vi "RSMA Receiver - 1 Channel 16QAM.vi"() -> ()   [LabVIEW 2022 SP3]
panel:
  out "Decoded message 2":string
  out "Acc. BER 2":dbl format="%#_4g"
  out "No. Bits 2":dbl format="%#_6f"
  out "Inst. BER 2":dbl format="%#_4g"
  out "Acum. Err 2":dbl
  in  "Expected message 2":string="rmod tempor invidunt ut labore et dolore magna aliquyam erat, sed diam volu"
  out "Number of bits":dbl[](array[numeric])
  out "Accuracy error":dbl[](array[numeric])
  out "Accumulated error":dbl[](array[numeric])
  out "Iterations":dbl format="%#_4g"
  out "Decoded message":string
  out "Constellation Map":cdb[](graph)
  in  "Decode M2?":bool
  in  "Tab Control":enum32{"USRP Parameters", "Rx Info", "BER"}(tab)
  in  "USRP ControledParameters":T1={"Active Antenna"="RX2", "Gain (dB)"=0.0, "Carrier Frequency"=2400000000.0, "IQ Rate"=2000000.0, "Active channels"="0"} {"IQ Rate" format="%#_6p"; "Carrier Frequency" format="%#_6p"; "Gain (dB)" format="%#_6f"}
  in  "Device selection":refnum<k15>="RIO0"
  in  "Trigger level":dbl=0.01 format="%f"
  out "?":T2
  out "SIG valid?":bool
  out "Frequency offset":dbl
  out "Coerced Parameters":T3={"IQ Rate"=100000.0, "Carrier  Freq."=100000.0, "Gain"=0.0} {"Gain" format="%#_6f"; "Carrier  Freq." format="%#_6p"; "IQ Rate" format="%#_6p"}
  out "Error out":errorcluster
  in  "Expected message":string="Lorem ipsum dolor sit amet, consetetur sadipscing elitr, sed diam nonumy eirmod tempor invidunt ut labore et dolore magna aliquyam erat, sed diam volu"
  in  "Record BER":bool
  in  "Refresh Button":bool
  out "Inst. BER":dbl format="%#_4g"
  out "No. Bits":dbl format="%#_6f"
  out "Acum. Err":dbl
  out "Acc. BER":dbl format="%#_4g"
  in  "error in (no error)":errorcluster
  # "RSMA Reciever"
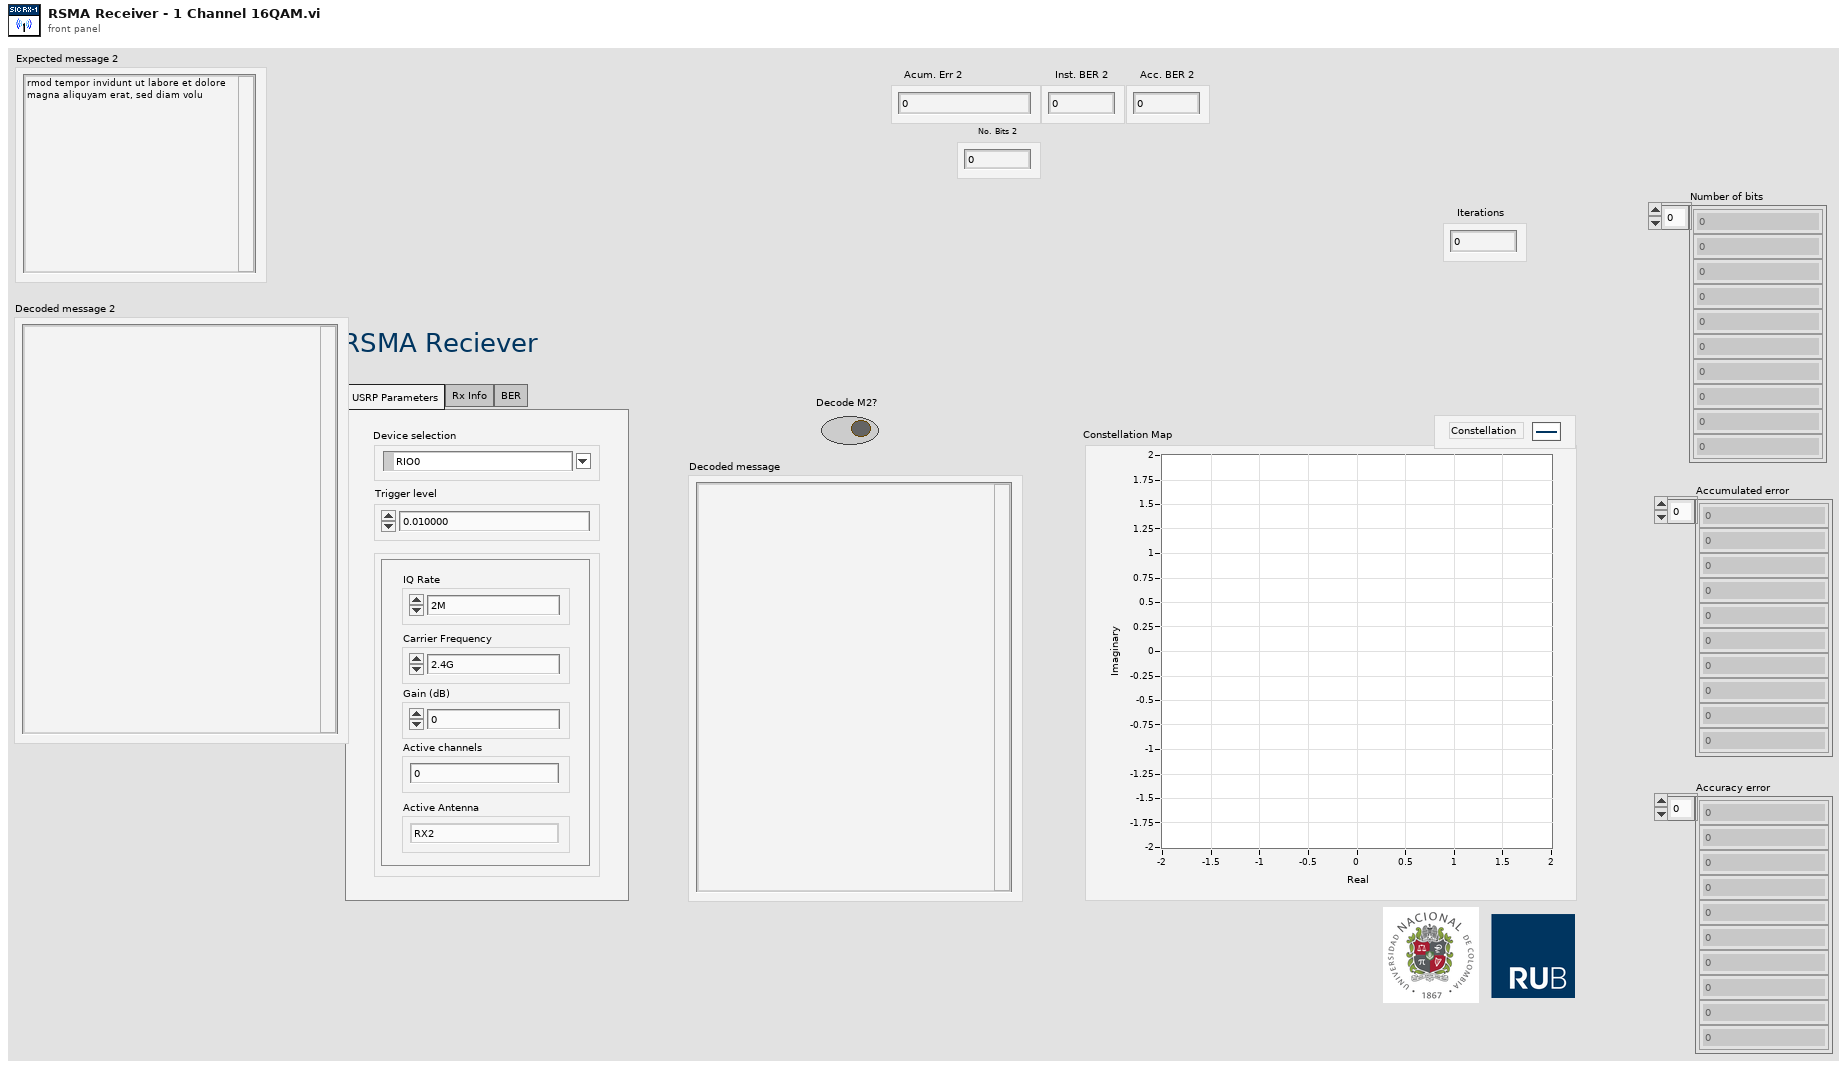
[diagram p1: front panel]
types:
  T1 = cluster{"Active Antenna":string, "Gain (dB)":dbl, "Carrier Frequency":dbl, "IQ Rate":dbl, "Active channels":string}
  T2 = cluster{"Modulation type":enum16{"QPSK(4QAM)", "64QAM", "16QAM", "BPSK"}, "BCC rate (k/n)":enum16{"1/2", "2/3", "3/4"}}
  T3 = cluster{"IQ Rate":dbl, "Carrier  Freq.":dbl, "Gain":dbl}
  T4 = cluster{"coerced IQ rate":dbl, "coerced carrier frequency":dbl, "coerced gain":dbl}
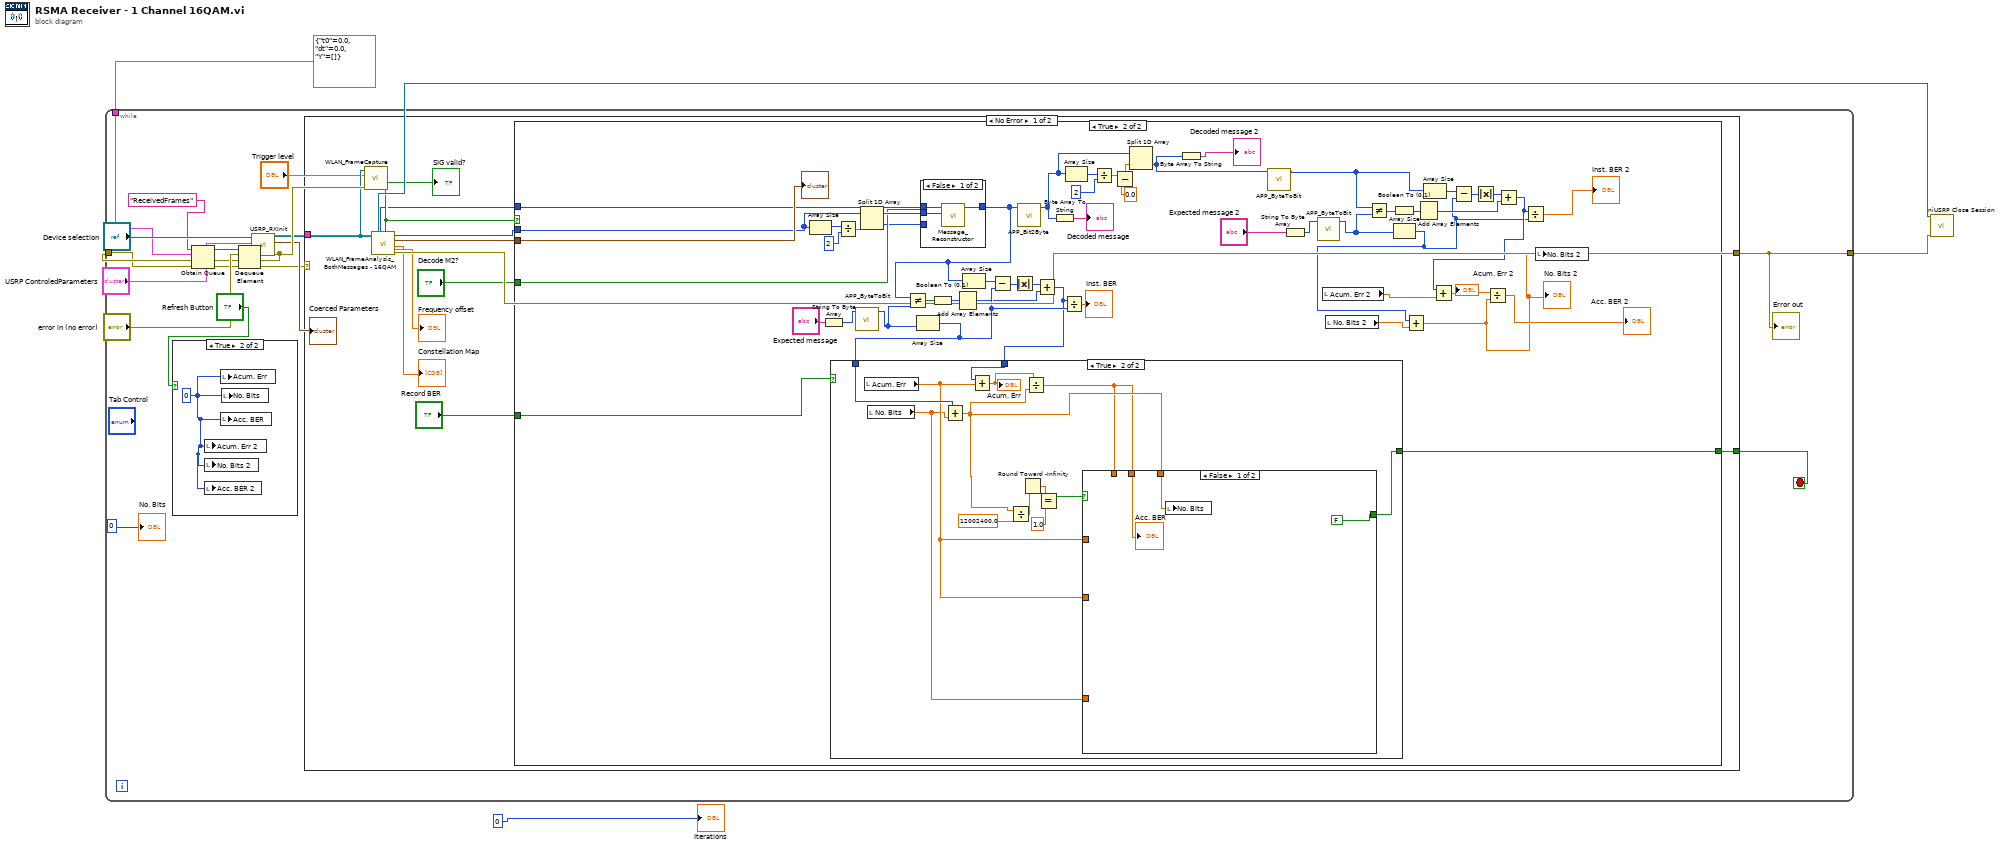
[diagram p0: block diagram]
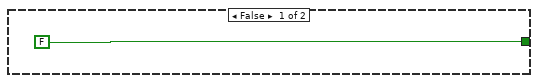
[diagram p3: hidden frame]
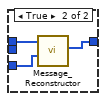
[diagram p4: hidden frame]
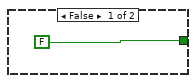
[diagram p5: hidden frame]
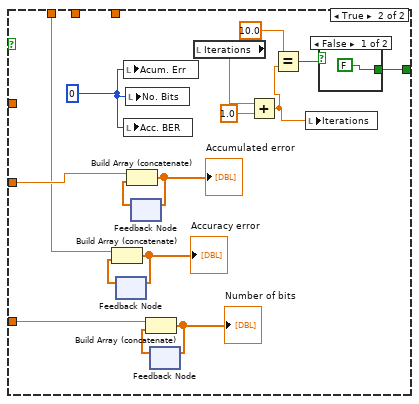
[diagram p6: hidden frame]
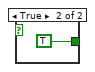
[diagram p7: hidden frame]
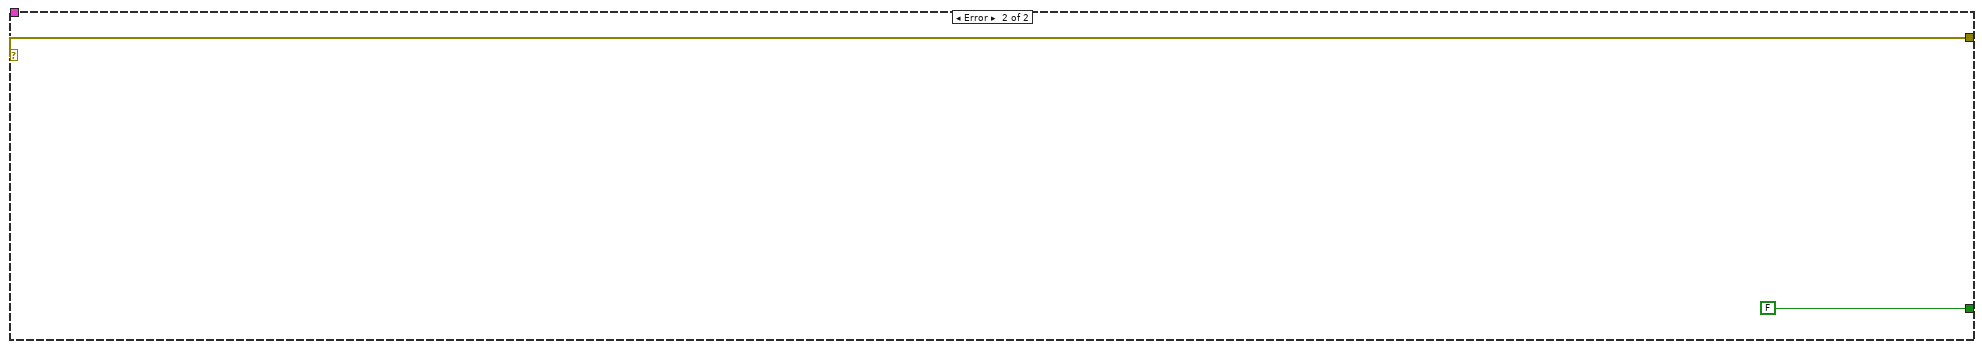
[diagram p8: hidden frame]
diagram:
  n1 = call "USRP_RXInit.vi"("device names"="Device selection", "USRP ControledParameters"="USRP ControledParameters", "error in (no error)"="error in (no error)") -> ("session handle out"=w7:refnum<k15>, "USRP CoercedParamters"=→"Coerced Parameters":T4, "error out"=w10:errorcluster)  [unwired: 5 in]
  n2 = while {
    tunnel: w10 -> [w20]
    tunnel: cluster{"t0":dbl, "dt":dbl, "Y":cdb[]} {"t0"=0.0, "dt"=0.0, "Y"=[]} ("data") -> [w21]
    tunnel: [w14] -> w8
    stop <- w12 stop-if-true
    n3 = case shown="True" "Refresh Button" {
      frame False {
      }
      frame True {
        w22 = 0
        n4 = local write "Acum. Err 2"(w22) -> ()
        n5 = local write "No. Bits 2"(w22) -> ()
        n6 = local write "Acc. BER 2"(w22) -> ()
        n7 = local write "Acum. Err"(w22) -> ()
        n8 = local write "Acc. BER"(w22) -> ()
        n9 = local write "No. Bits"(w22) -> ()
      }
    }
    n10 = Obtain Queue(name (unnamed)="ReceivedFrames", element data type=w21, error in (no error)=w20) -> (queue out=w19:refnum<queue>, error out=w16:errorcluster)  [unwired: 2 in, 1 out]
    n11 = Dequeue Element(queue=w19, error in (no error)=w16) -> (element=w17:cluster{"t0":dbl, "dt":dbl, "Y":cdb[]}, error out=w18:errorcluster)  [unwired: 1 in, 2 out]
    n12 = case shown="No Error" w18 {
      selector: w18 -> [_ w128]
      tunnel: w17 -> [w31 _]
      tunnel: [w32 w128] -> w14
      tunnel: [w23 FALSE] -> w12
      frame No Error {
        n13 = call "WLAN_FrameAnalysis_BothMessages - 16QAM.vi"("input cluster"=w31) -> ("error out"=w32:errorcluster, "Constellation"=→"Constellation Map":cdb[], "Modulation parameter"=w33:T2, "SC Bits"=w25:i8[], "Frequency offset"=→"Frequency offset":dbl, "SIG valid?"=w30:bool, "Base Bits"=w26:i8[])  [unwired: 4 in]
        "SIG valid?" <- w30
        n14 = case shown="True" w30 {
          tunnel: w33 -> [_ w85]
          tunnel: "Record BER" -> [_ w79]
          tunnel: w26 -> [_ w67]
          tunnel: w25 -> [_ w63]
          tunnel: "Decode M2?" -> [_ w66]
          tunnel: [FALSE w62] -> w23
          frame False {
          }
          frame True {
            n15 = Array Size(array=w63) -> (size(s)=w69:i32)
            n16 = String To Byte Array(string="Expected message") -> (unsigned byte array=w78:u8[])
            n17 = Divide(x=w69, y=2) -> (x/y=w70:dbl)
            n18 = call "APP_ByteToBit.vi"("byte array"=w78) -> ("bit array"=w77:i8[])  [unwired: 9 in]
            n19 = Split 1D Array(array=w63, index=w70) -> (first subarray=w68:i8[], second subarray=w65:i8[])
            n20 = Array Size(array=w77) -> (size(s)=w73:i32)
            n21 = case shown="False" w66 {
              tunnel: [w88 w89] -> w43
              tunnel: w68 -> [w87 _]
              tunnel: w67 -> [w86 w90]
              tunnel: w65 -> [_ w91]
              frame False {
                n22 = call "Message_Reconstructor.vi"("Wp1"=w87, "Wc"=w86) -> ("W1"=w88:u8[])  [unwired: 8 in, 1 out]
              }
              frame True {
                n23 = call "Message_Reconstructor.vi"("Wp2"=w91, "Wc"=w90) -> ("W2"=w89:u8[])  [unwired: 8 in, 1 out]
              }
            }
            n24 = Not Equal?(x=w43, y=w77) -> (x != y?=w81:bool[])
            n25 = Boolean To (0,1)(Boolean=w81) -> (0, 1=w80:i16[])
            n26 = Add Array Elements(numeric array=w80) -> (sum=w72:i16)
            n27 = Array Size(array=w43) -> (size(s)=w76:i32)
            n28 = Subtract(x=w76, y=w73) -> (x-y=w75:i32)
            n29 = Absolute Value(x=w75) -> (abs(x)=w74:i32)
            n30 = call "APP_Bit2Byte.vi"("input bit stream"=w43) -> ("output byte stream"=w45:u8[])  [unwired: 10 in]
            n31 = Add(x=w74, y=w72) -> (x+y=w71:i32)
            n32 = case shown="True" w79 {
              tunnel: w73 -> [_ w105]
              tunnel: w71 -> [_ w104]
              tunnel: [FALSE w96] -> w62
              frame False {
              }
              frame True {
                n33 = local read "Acum. Err"() -> (w95:dbl)
                n34 = local read "No. Bits"() -> (w93:dbl)
                n35 = Add(x=w105, y=w93) -> (x+y=w99:dbl)
                n36 = Add(x=w104, y=w95) -> (x+y=w103:dbl)
                "Acum. Err" <- w103
                n37 = Divide(x=w99, y=12002400.0) -> (x/y=w98:dbl)
                n38 = Round Toward -Infinity(1:w98) -> (0:w97:dbl)
                n39 = Divide(x=w103, y=w99) -> (x/y=w94:dbl)
                n40 = Equal?(x=w97, y=1.0) -> (x = y?=w100:bool)
                n41 = case shown="False" w100 {
                  tunnel: w95 -> [_ _]
                  tunnel: w99 -> [w108 _]
                  tunnel: w94 -> [w107 _]
                  tunnel: [FALSE w119] -> w96
                  tunnel: w95 -> [_ w117]
                  tunnel: w94 -> [_ w112]
                  tunnel: w93 -> [_ w109]
                  frame False {
                    n42 = local write "No. Bits"(w108) -> ()
                    "Acc. BER" <- w107
                  }
                  frame True {
                    w124 = 0
                    n43 = feedback #1() -> (w114:dbl[])  [unwired: 1 in]
                    n44 = Build Array (concatenate)(w112, w114) -> (w113:dbl[])
                    "Accuracy error" <- w113
                    n45 = feedback-in #1(w113) -> ()
                    n46 = local write "Acum. Err"(w124) -> ()
                    n47 = local write "Acc. BER"(w124) -> ()
                    n48 = local write "No. Bits"(w124) -> ()
                    n49 = feedback #2() -> (w116:dbl[])  [unwired: 1 in]
                    n50 = Build Array (concatenate)(w117, w116) -> (w115:dbl[])
                    "Accumulated error" <- w115
                    n51 = feedback-in #2(w115) -> ()
                    n52 = feedback #3() -> (w111:dbl[])  [unwired: 1 in]
                    n53 = Build Array (concatenate)(w109, w111) -> (w110:dbl[])
                    "Number of bits" <- w110
                    n54 = feedback-in #3(w110) -> ()
                    n55 = local read "Iterations"() -> (w123:dbl)
                    n56 = Add(x=w123, y=1.0) -> (x+y=w118:dbl)
                    n57 = Equal?(x=10.0, y=w118) -> (x = y?=w120:bool)
                    n58 = local write "Iterations"(w118) -> ()
                    n59 = case shown="False" w120 {
                      tunnel: [FALSE TRUE] -> w119
                      frame False {
                      }
                      frame True {
                      }
                    }
                  }
                }
              }
            }
            n60 = Byte Array To String(unsigned byte array=w45) -> (string=→"Decoded message":string)
            n61 = Divide(x=w71, y=w73) -> (x/y=→"Inst. BER":dbl)
            n62 = Array Size(array=w45) -> (size(s)=w46:i32)
            n63 = Divide(x=w46, y=2) -> (x/y=w40:dbl)
            n64 = Subtract(x=w40, y=0.0) -> (x-y=w38:dbl)
            n65 = Split 1D Array(array=w45, index=w38) -> (second subarray=w37:u8[])  [unwired: 1 out]
            n66 = Byte Array To String(unsigned byte array=w37) -> (string=→"Decoded message 2":string)
            n67 = call "APP_ByteToBit.vi"("byte array"=w37) -> ("bit array"=w36:i8[])  [unwired: 9 in]
            n68 = String To Byte Array(string="Expected message 2") -> (unsigned byte array=w59:u8[])
            n69 = call "APP_ByteToBit.vi"("byte array"=w59) -> ("bit array"=w35:i8[])  [unwired: 9 in]
            n70 = local read "Acum. Err 2"() -> (w56:dbl)
            n71 = local read "No. Bits 2"() -> (w55:dbl)
            n72 = Not Equal?(x=w36, y=w35) -> (x != y?=w58:bool[])
            n73 = Boolean To (0,1)(Boolean=w58) -> (0, 1=w57:i16[])
            n74 = Array Size(array=w35) -> (size(s)=w51:i32)
            n75 = Add(x=w51, y=w55) -> (x+y=w41:dbl)
            "No. Bits 2" <- w41
            n76 = Add Array Elements(numeric array=w57) -> (sum=w61:i16)
            n77 = Array Size(array=w36) -> (size(s)=w44:i32)
            n78 = Subtract(x=w44, y=w51) -> (x-y=w54:i32)
            n79 = Absolute Value(x=w54) -> (abs(x)=w53:i32)
            n80 = Add(x=w53, y=w61) -> (x+y=w52:i32)
            n81 = Add(x=w52, y=w56) -> (x+y=w50:dbl)
            "Acum. Err 2" <- w50
            n82 = Divide(x=w50, y=w41) -> (x/y=→"Acc. BER 2":dbl)
            n83 = Divide(x=w52, y=w51) -> (x/y=→"Inst. BER 2":dbl)
            n84 = local write "No. Bits 2"(w41) -> ()
            "?" <- w85
          }
        }
      }
      frame Error {
      }
    }
    "Error out" <- w14
  }
  n85 = call "WLAN_FrameCapture.vi"("error in (no error)"=w10, "Trigger level"="Trigger level", "session handle"=w7) -> ()  [unwired: 8 in]
  n86 = call <instrlib>:"niUSRP Close Session.vi"("session handle"=w7, "error in (no error)"=w8) -> ()  [unwired: 13 in, 1 out]
  "No. Bits" <- 0
  "Iterations" <- 0
